vi "挥发酚通讯.vi"() -> ()   [LabVIEW 2022 SP3, in "挥发酚.lvlib"]
uses:
  <vilib>/Utility/config.llb/Write Key (String).vi
  <vilib>/Plasmionique/MB Master/MB_Master/MB_Master.lvclass
  <vilib>/Utility/config.llb/NI_LVConfig.lvlib
  <vilib>/Plasmionique/MB Master/MB Master.lvlib
  <userlib>/_OpenG.lib/variantconfig/variantconfig.llb/openg_variant_configuration_file.lvlib
  <vilib>/ptbypt/NI_PtbyPt.lvlib
panel:
  out "状态告警区":T1 {"工作状态" items=["空闲"=0, "水样测试"=1, "标样核查"=2, "零点核查"=3, "跨度核查"=4, "空白测试"=5, "平行样测试"=6, "加标回收"=7, "空白校准"=8, "标样校准"=9, "标定"=19, "初始化（清洗）"=10, "标样1测量"=28, "标样2测量"=29, "故障"=30, "异常处理"=31, "初始装液"=32, "其他"=33]; "告警代码" items=["无告警", "缺试剂告警", "缺水样告警", "缺蒸馏水告警", "缺标液告警", "仪表漏液告警", "标定异常告警", "超量程告警", "加热异常", "低试剂预警", "超上限告警", "超下限告警", "仪表内部其他异常", "滴定异常告警", "电极异常告警", "量程切换告警", "参数设置告警", "PH电极电位异常", "电导率电极异常", "浊度光度异常", "溶解氧电极异常", "溶解氧光强异常", "温度异常告警", "PH异常告警", "溶解氧异常告警", "电导率异常告警", "浊度异常告警", "叶绿素异常告警", "藻密度异常告警", "蓝绿藻异常告警", "ORP异常告警", "氨氮异常告警", "清洁刷异常告警", "SD卡异常告警", "蓝牙异常告警", "Wifi异常告警", "流程异常告警"]; "故障代码" items=["无故障", "电机故障", "温度故障", "通讯故障", "滴定故障"]}
  out "控制命令 2":u16[](array[numeric]) format="%xH"
  out "测量数据区":T2 {"单位" items=["ug/L", "mg/L", "ppm", "mg/m3", "cm", "ppb", "ug/m3", "%", "nmol/mol", "umol/mol", "MPN/L", "MPN/100ml", "ng/m3", "NTU", "无量纲", "ms/cm", "us/cm", "℃", "mV", "万个/L"]}
  out "状态告警区":u16[](array[numeric])
  out "测量数据区":u16[](array[numeric])
  out "序列号":string
  out "status":bool
  out "关键参数区":T3
  in  "读关键参数区":bool
  in  "读状态告警区":bool
  in  "读测量数据区":bool
  in  "站号":u16(ring) items=["CODMn"=21, "氨氮"=3, "挥发酚"=1]
  in  "停止":bool
  in  "启动":bool
  in  "控制命令":u16(ring) items=["启动测量"=1, "标样核查"=2, "零点核查"=3, "跨度核查"=4, "空白测试"=5, "平行样测试"=6, "加标回收"=7, "空白校准"=8, "标样校准"=9, "初始化（清洗）"=10, "停止测试"=11, "仪器重启"=12, "校时"=13, "模式设置"=14, "测量间隔设置"=15]
  in  "控制命令参数":u16[](array[numeric]) format="%04xH"
  in  "VISA Resource":refnum<visa-resource-name>
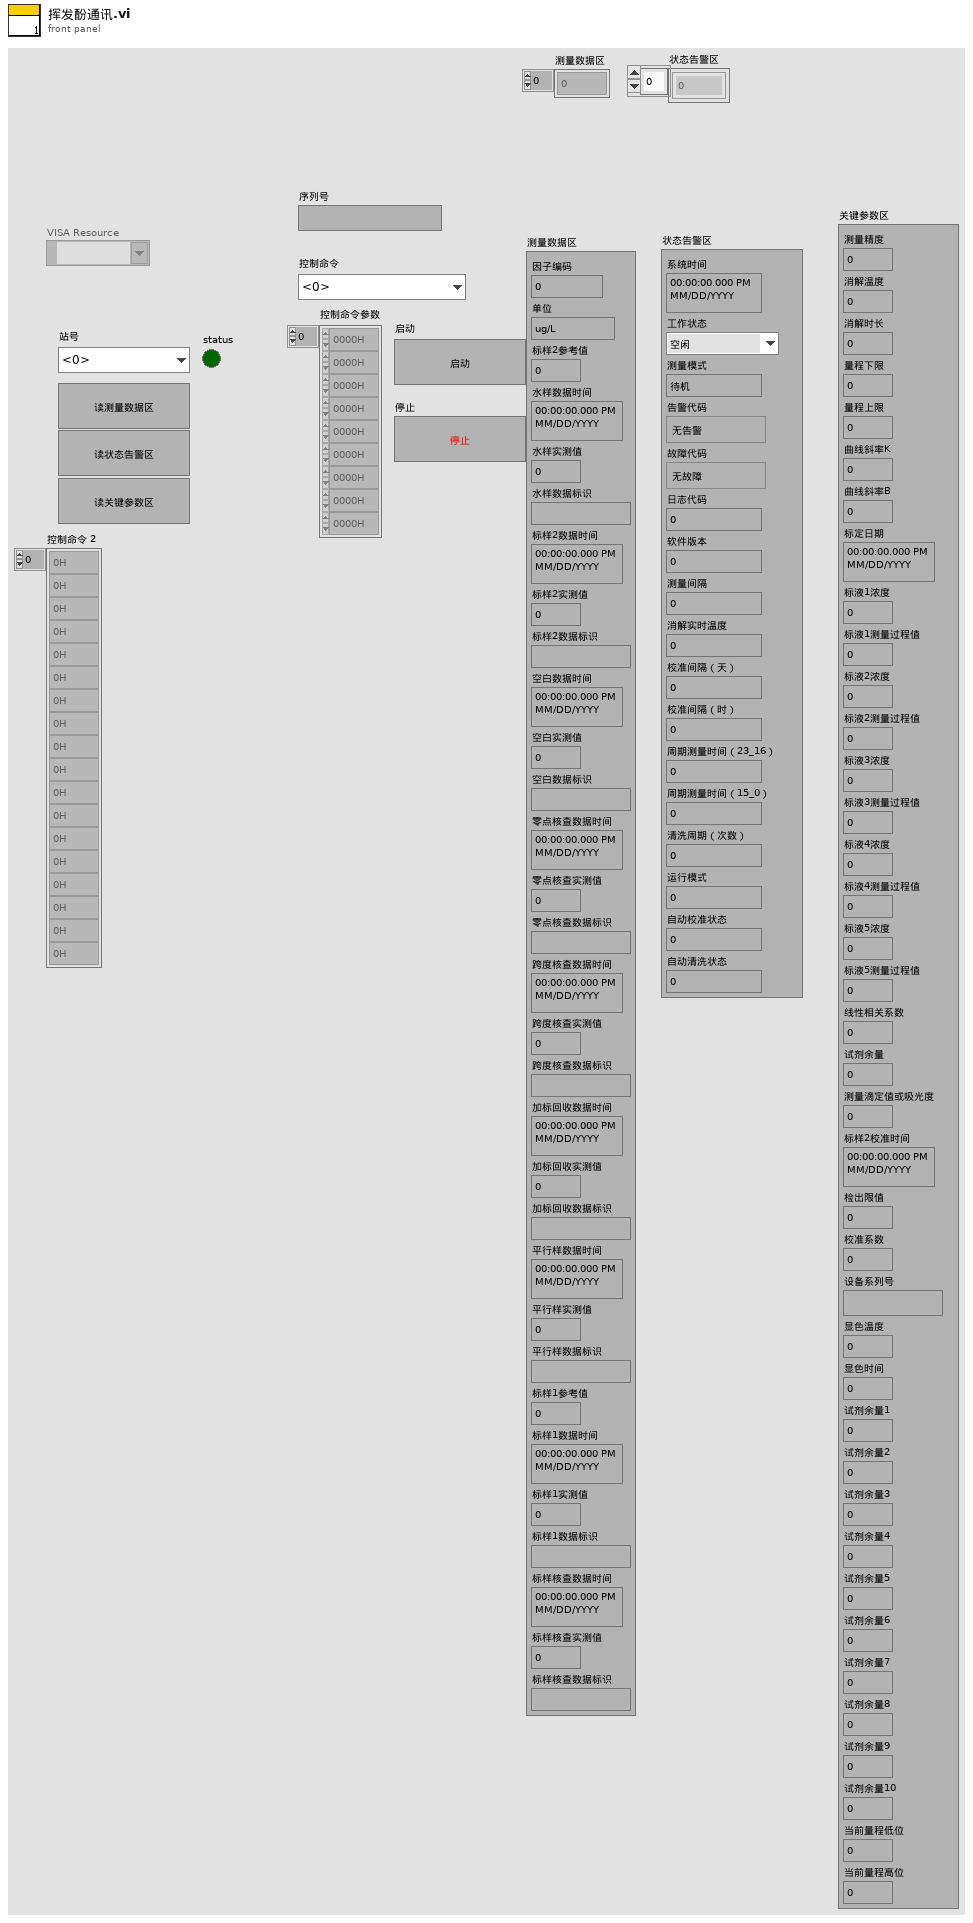
[diagram p1: front panel]
types:
  T1 = cluster{"系统时间":timestamp, "工作状态":u16, "测量模式":enum16{"待机", "连续模式", "周期模式", "定点模式", "受控模式", "手动模式"}, "告警代码":u16, "故障代码":u16, "日志代码":u16, "软件版本":u16, "测量间隔":u16, "消解实时温度":dbl, "校准间隔（天）":u16, "校准间隔（时）":u16, "周期测量时间（23_16）":u16, "周期测量时间（15_0）":u16, "清洗周期（次数）":u16, "运行模式":u16, "自动校准状态":u16, "自动清洗状态":u16}
  T2 = cluster{"因子编码":u32, "单位":u16, "标样2参考值":sgl, "水样数据时间":timestamp, "水样实测值":sgl, "水样数据标识":string, "标样2数据时间":timestamp, "标样2实测值":sgl, "标样2数据标识":string, "空白数据时间":timestamp, "空白实测值":sgl, "空白数据标识":string, "零点核查数据时间":timestamp, "零点核查实测值":sgl, "零点核查数据标识":string, "跨度核查数据时间":timestamp, "跨度核查实测值":sgl, "跨度核查数据标识":string, "加标回收数据时间":timestamp, "加标回收实测值":sgl, "加标回收数据标识":string, "平行样数据时间":timestamp, "平行样实测值":sgl, "平行样数据标识":string, "标样1参考值":sgl, "标样1数据时间":timestamp, "标样1实测值":sgl, "标样1数据标识":string, "标样核查数据时间":timestamp, "标样核查实测值":sgl, "标样核查数据标识":string}
  T3 = cluster{"测量精度":u16, "消解温度":u16, "消解时长":u16, "量程下限":sgl, "量程上限":sgl, "曲线斜率K":sgl, "曲线斜率B":sgl, "标定日期":timestamp, "标液1浓度":sgl, "标液1测量过程值":sgl, "标液2浓度":sgl, "标液2测量过程值":sgl, "标液3浓度":sgl, "标液3测量过程值":sgl, "标液4浓度":sgl, "标液4测量过程值":sgl, "标液5浓度":sgl, "标液5测量过程值":sgl, "线性相关系数":sgl, "试剂余量":u32, "测量滴定值或吸光度":sgl, "标样2校准时间":timestamp, "检出限值":sgl, "校准系数":sgl, "设备系列号":string, "显色温度":u16, "显色时间":u16, "试剂余量1":u16, "试剂余量2":u16, "试剂余量3":u16, "试剂余量4":u16, "试剂余量5":u16, "试剂余量6":u16, "试剂余量7":u16, "试剂余量8":u16, "试剂余量9":u16, "试剂余量10":u16, "当前量程低位":sgl, "当前量程高位":sgl}
  T4 = cluster{"测量模式":enum16{"水样测量", "标样核查", "零点核查", "跨度核查", "空白测试", "加标回收", "平行样", "校零", "校标"}}
  T5 = typedef "NI_LVConfig.lvlib/Config Data RefNum.ctl" = refnum<k1>
  T6 = cluster{"站号":u16, "量程切换":enum32{"H", "L", "AUTO"}, "控制命令":u16, "模式设置":enum16{"待机", "连续模式", "周期模式", "定点模式", "受控模式", "手动模式"}, "测量间隔":u16}
  T7 = enum16{"水样测量", "标样核查", "零点核查", "跨度核查", "空白测试", "加标回收", "平行样", "校零", "校标"}
  T8 = enum8{"Enabled", "Disabled", "Disabled and Grayed Out"}
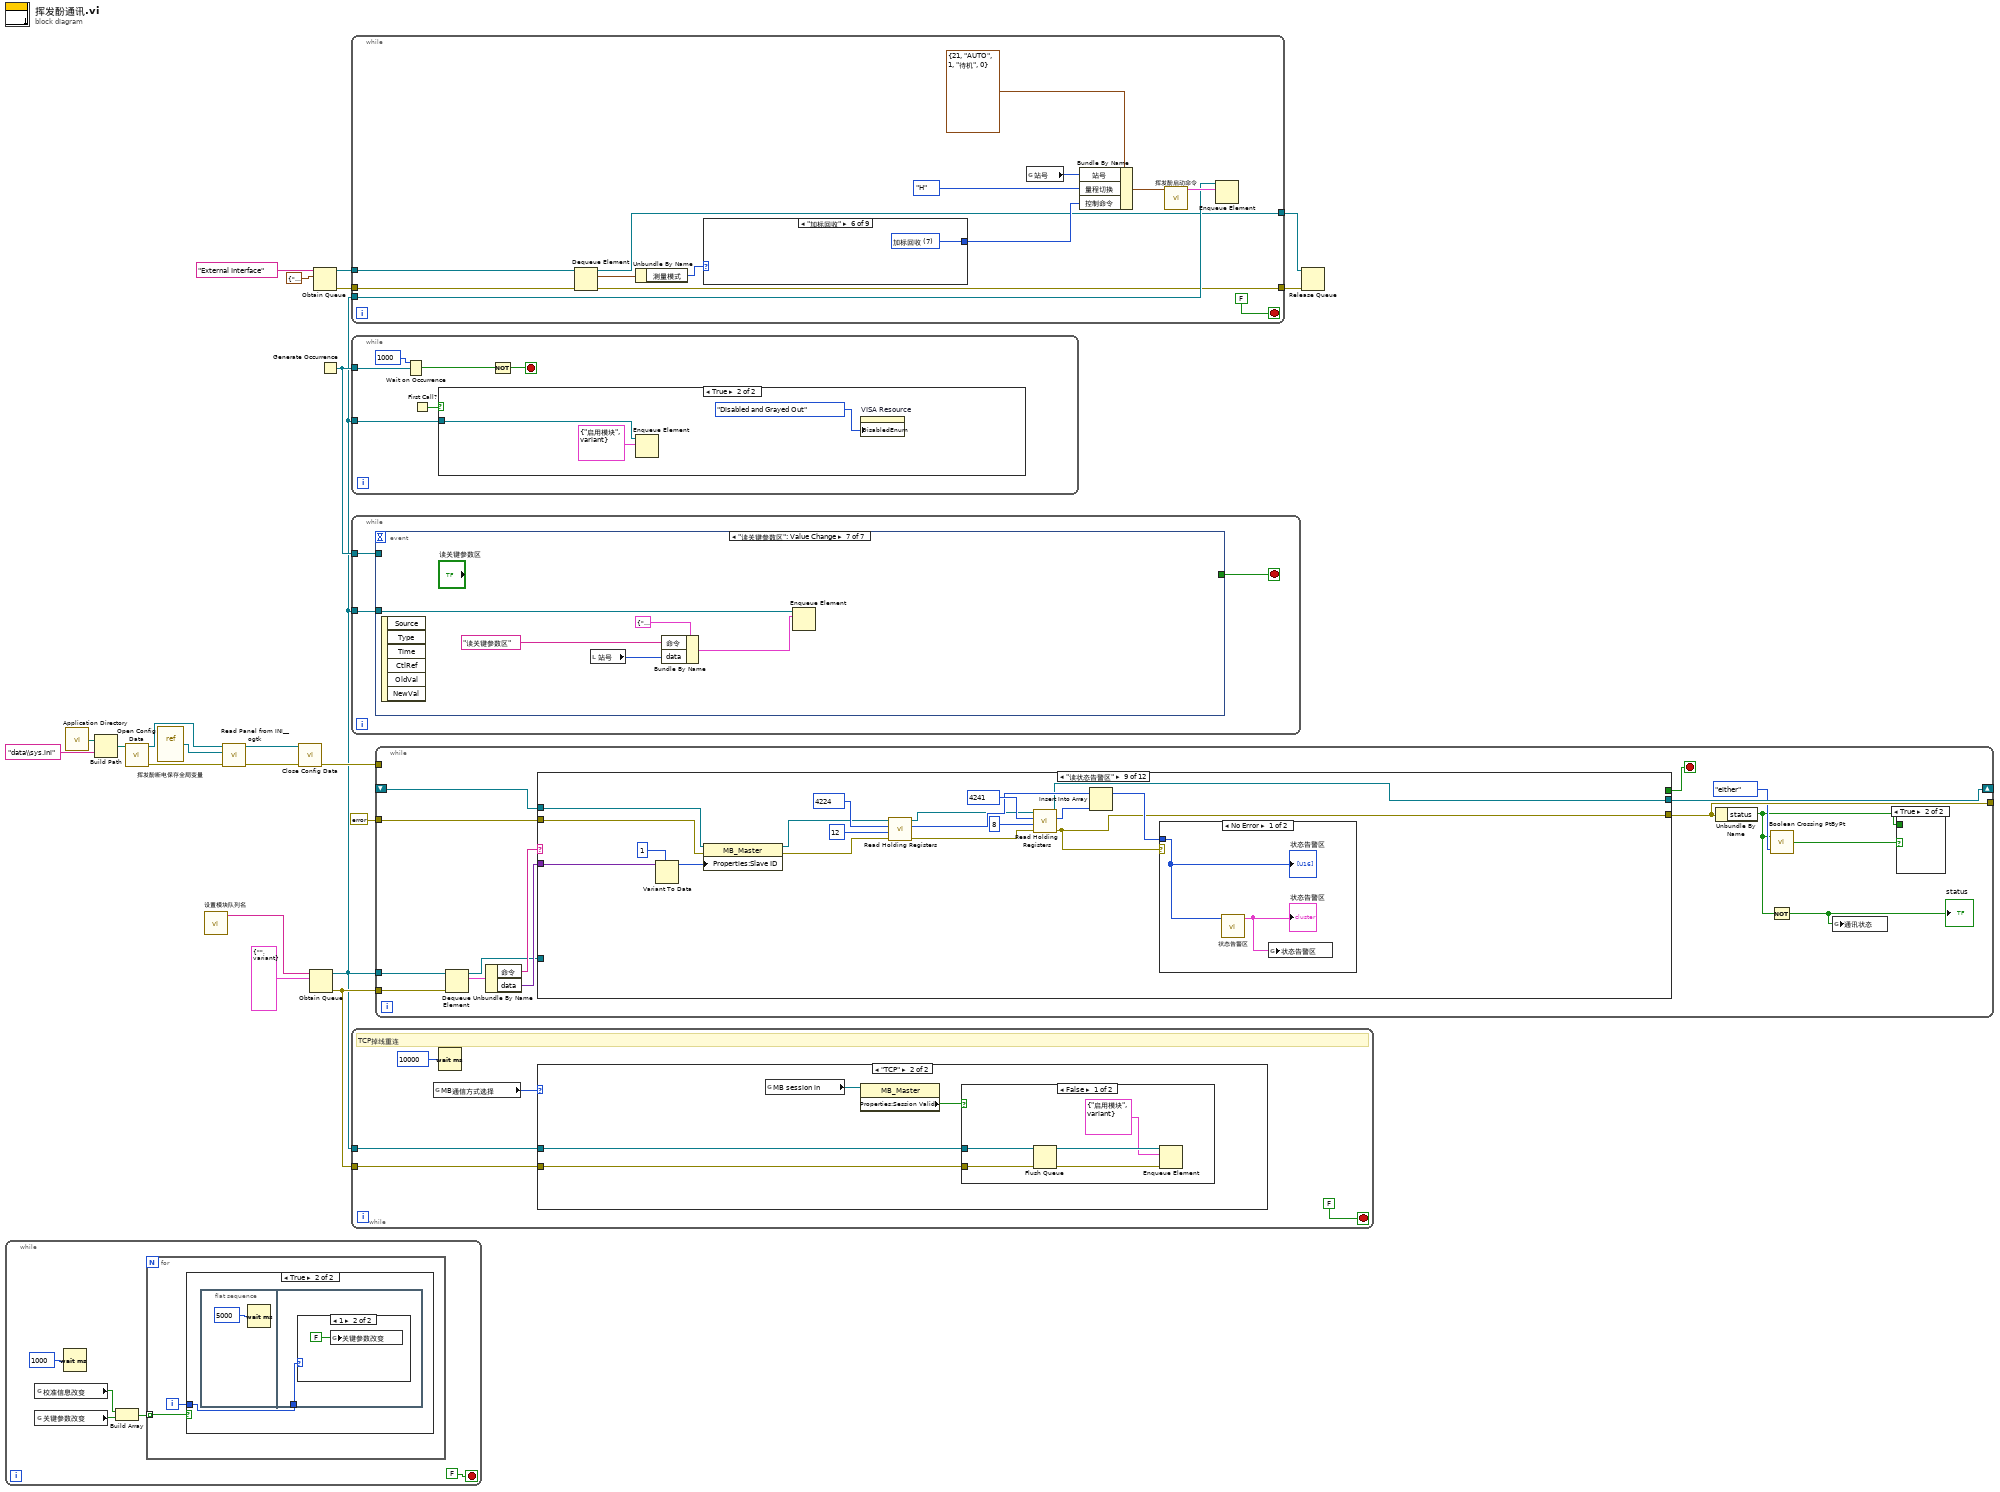
[diagram p0: block diagram]
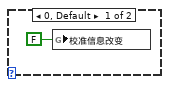
[diagram p3: hidden frame]
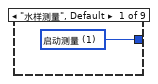
[diagram p4: hidden frame]
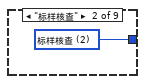
[diagram p5: hidden frame]
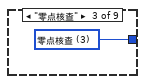
[diagram p6: hidden frame]
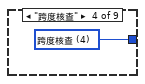
[diagram p7: hidden frame]
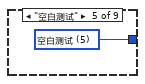
[diagram p8: hidden frame]
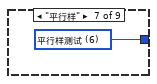
[diagram p9: hidden frame]
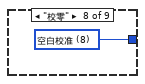
[diagram p10: hidden frame]
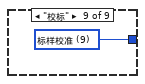
[diagram p11: hidden frame]
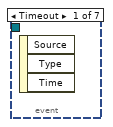
[diagram p15: hidden frame]
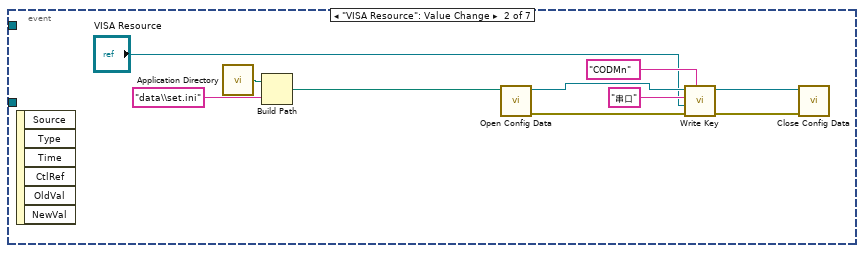
[diagram p16: hidden frame]
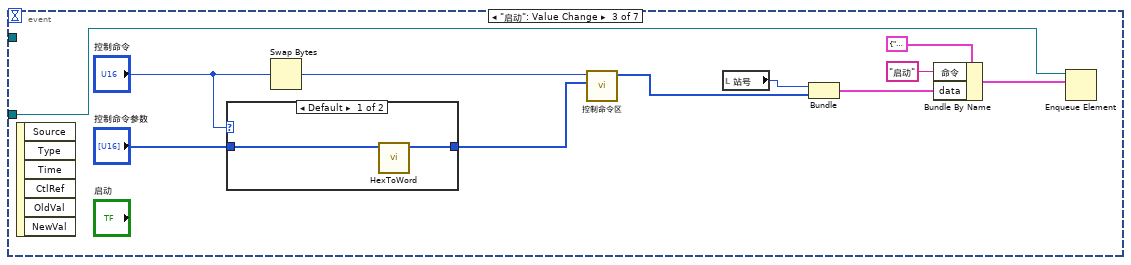
[diagram p17: hidden frame]
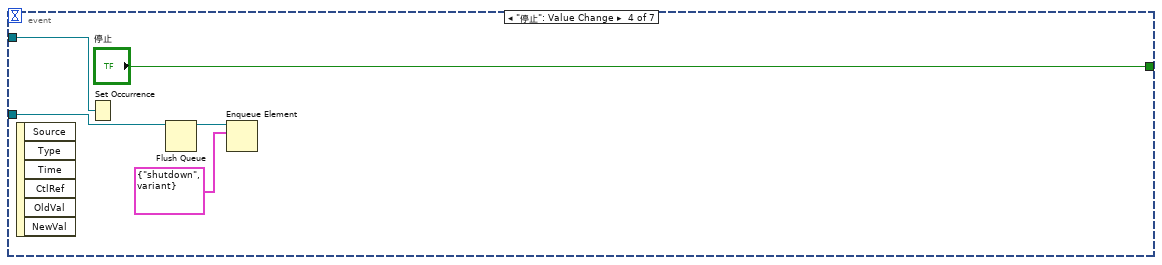
[diagram p19: hidden frame]
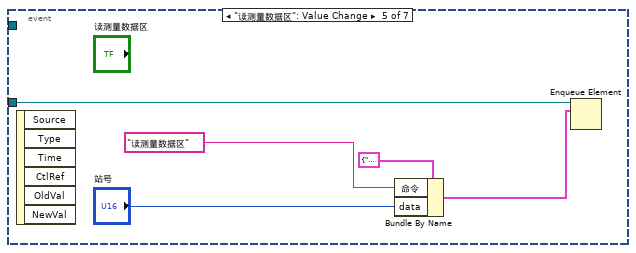
[diagram p20: hidden frame]
diagram:
  n1 = while {
    stop <- FALSE stop-if-true
    n2 = global read "挥发酚断电保存全局变量.vi" "校准信息改变"() -> (w24:bool)
    n3 = global read "挥发酚断电保存全局变量.vi" "关键参数改变"() -> (w23:bool)
    n4 = Wait (ms)(milliseconds to wait=u32 1000 ("等待时间（毫秒）")) -> ()  [unwired: 1 out]
    n5 = Build Array(w24, w23) -> (w22:bool[])
    n6 = for {
      tunnel: w22 -> [w28] mode=indexing
      i -> [w27]
      n7 = case shown="True" w28 {
        tunnel: w27 -> [_ w29]
        frame False {
        }
        frame True {
          n8 = flat-sequence {
            tunnel: w29 -> [w31]
            frame #0 {
              n9 = Wait (ms)(milliseconds to wait=u32 5000 ("等待时间（毫秒）")) -> ()  [unwired: 1 out]
            }
            frame #1 {
              n10 = case shown="1" w31 {
                frame 0, Default {
                  n11 = global write "挥发酚断电保存全局变量.vi" "校准信息改变"(FALSE ("关键参数改变")) -> ()
                }
                frame 1 {
                  n12 = global write "挥发酚断电保存全局变量.vi" "关键参数改变"(FALSE ("关键参数改变")) -> ()
                }
              }
            }
          }
        }
      }
    }
  }
  n13 = call <vilib>:"Application Directory.vi"() -> ("Application Directory"=w2:path)
  n14 = Build Path(base path=w2, name or relative path="data\\sys.ini" ("名称或相对路径")) -> (appended path=w11:path)
  n15 = call <vilib>:"Open Config Data.vi"("configuration file path"=w11) -> ("error out"=w17:errorcluster, "refnum"=w14:T5)  [unwired: 8 in, 1 out]
  n16 = vi-ref "挥发酚断电保存全局变量.vi"() -> (w15:refnum<vi>)
  n17 = call "设置模块队列名.vi"() -> ("Msg"=w3:string)  [unwired: 11 in]
  n18 = call <userlib>:"Read Panel from INI__ogtk.vi"("error in (no error)"=w17, "VI ref"=w15, "refnum"=w14) -> ("error out"=w18:errorcluster, "refnum out"=w16:T5)  [unwired: 7 in]
  n19 = call <vilib>:"Close Config Data.vi"("error in (no error)"=w18, "refnum"=w16) -> ("error out"=w13:errorcluster)  [unwired: 8 in, 1 out]
  n20 = Obtain Queue(name (unnamed)=w3, element data type=cluster{"命令":string, "data":variant} {"命令"="", "data"=variant}) -> (queue out=w7:refnum<queue>, error out=w12:errorcluster)  [unwired: 3 in, 1 out]
  n21 = Obtain Queue(name (unnamed)="External Interface" ("名称（未命名）"), element data type=T4 {"测量模式"=enum."水样测量"} ("元素")) -> (queue out=w9:refnum<queue>, error out=w8:errorcluster)  [unwired: 3 in, 1 out]
  n22 = Generate Occurrence() -> (w19:refnum<k4>)
  n23 = while {
    tunnel: w9 -> [w47]
    tunnel: w8 -> [w46]
    tunnel: w7 -> [w38]
    tunnel: [w37] -> w6
    tunnel: [w36] -> w5
    stop <- FALSE stop-if-true
    n24 = Dequeue Element(queue=w47, error in (no error)=w46) -> (queue out=w37:refnum<queue>, element=w41:T4, error out=w36:errorcluster)  [unwired: 1 in, 1 out]
    n25 = Unbundle By Name(w41) -> ("测量模式"=w40:T7)
    n26 = case shown="\"加标回收\"" w40 {
      tunnel: [w48 w49 w50 w51 w52 w53 w54 w55 w56] -> w39
      frame "水样测量", Default {
        w48 = u16 1 items=["启动测量"=1, "标样核查"=2, "零点核查"=3, "跨度核查"=4, "空白测试"=5, "平行样测试"=6, "加标回收"=7, "空白校准"=8, "标样校准"=9, "初始化（清洗）"=10, "停止测试"=11, "仪器重启"=12, "校时"=13, "模式设置"=14, "测量间隔设置"=15, "调试"=22, "填充管路"=30, "清洗管路"=31, "清洗反应杯"=32] ("控制命令")
      }
      frame "标样核查" {
        w49 = u16 2 items=["启动测量"=1, "标样核查"=2, "零点核查"=3, "跨度核查"=4, "空白测试"=5, "平行样测试"=6, "加标回收"=7, "空白校准"=8, "标样校准"=9, "初始化（清洗）"=10, "停止测试"=11, "仪器重启"=12, "校时"=13, "模式设置"=14, "测量间隔设置"=15, "调试"=22, "填充管路"=30, "清洗管路"=31, "清洗反应杯"=32] ("控制命令")
      }
      frame "零点核查" {
        w50 = u16 3 items=["启动测量"=1, "标样核查"=2, "零点核查"=3, "跨度核查"=4, "空白测试"=5, "平行样测试"=6, "加标回收"=7, "空白校准"=8, "标样校准"=9, "初始化（清洗）"=10, "停止测试"=11, "仪器重启"=12, "校时"=13, "模式设置"=14, "测量间隔设置"=15, "调试"=22, "填充管路"=30, "清洗管路"=31, "清洗反应杯"=32] ("控制命令")
      }
      frame "跨度核查" {
        w51 = u16 4 items=["启动测量"=1, "标样核查"=2, "零点核查"=3, "跨度核查"=4, "空白测试"=5, "平行样测试"=6, "加标回收"=7, "空白校准"=8, "标样校准"=9, "初始化（清洗）"=10, "停止测试"=11, "仪器重启"=12, "校时"=13, "模式设置"=14, "测量间隔设置"=15, "调试"=22, "填充管路"=30, "清洗管路"=31, "清洗反应杯"=32] ("控制命令")
      }
      frame "空白测试" {
        w52 = u16 5 items=["启动测量"=1, "标样核查"=2, "零点核查"=3, "跨度核查"=4, "空白测试"=5, "平行样测试"=6, "加标回收"=7, "空白校准"=8, "标样校准"=9, "初始化（清洗）"=10, "停止测试"=11, "仪器重启"=12, "校时"=13, "模式设置"=14, "测量间隔设置"=15, "调试"=22, "填充管路"=30, "清洗管路"=31, "清洗反应杯"=32] ("控制命令")
      }
      frame "加标回收" {
        w53 = u16 7 items=["启动测量"=1, "标样核查"=2, "零点核查"=3, "跨度核查"=4, "空白测试"=5, "平行样测试"=6, "加标回收"=7, "空白校准"=8, "标样校准"=9, "初始化（清洗）"=10, "停止测试"=11, "仪器重启"=12, "校时"=13, "模式设置"=14, "测量间隔设置"=15, "调试"=22, "填充管路"=30, "清洗管路"=31, "清洗反应杯"=32] ("控制命令")
      }
      frame "平行样" {
        w54 = u16 6 items=["启动测量"=1, "标样核查"=2, "零点核查"=3, "跨度核查"=4, "空白测试"=5, "平行样测试"=6, "加标回收"=7, "空白校准"=8, "标样校准"=9, "初始化（清洗）"=10, "停止测试"=11, "仪器重启"=12, "校时"=13, "模式设置"=14, "测量间隔设置"=15, "调试"=22, "填充管路"=30, "清洗管路"=31, "清洗反应杯"=32] ("控制命令")
      }
      frame "校零" {
        w55 = u16 8 items=["启动测量"=1, "标样核查"=2, "零点核查"=3, "跨度核查"=4, "空白测试"=5, "平行样测试"=6, "加标回收"=7, "空白校准"=8, "标样校准"=9, "初始化（清洗）"=10, "停止测试"=11, "仪器重启"=12, "校时"=13, "模式设置"=14, "测量间隔设置"=15, "调试"=22, "填充管路"=30, "清洗管路"=31, "清洗反应杯"=32] ("控制命令")
      }
      frame "校标" {
        w56 = u16 9 items=["启动测量"=1, "标样核查"=2, "零点核查"=3, "跨度核查"=4, "空白测试"=5, "平行样测试"=6, "加标回收"=7, "空白校准"=8, "标样校准"=9, "初始化（清洗）"=10, "停止测试"=11, "仪器重启"=12, "校时"=13, "模式设置"=14, "测量间隔设置"=15, "调试"=22, "填充管路"=30, "清洗管路"=31, "清洗反应杯"=32] ("控制命令")
      }
    }
    n27 = global read "挥发酚断电保存全局变量.vi" "站号"() -> (w42:u16)
    n28 = Bundle By Name(cluster=T6 {"站号"=21, "量程切换"=enum."AUTO", "控制命令"=1, "模式设置"=enum."待机", "测量间隔"=0} ("参数"), "站号"=w42, "量程切换"=enum32{"H", "L", "AUTO"}."H", "控制命令"=w39) -> (w43:T6)
    n29 = call "挥发酚启动命令.vi"("参数"=w43) -> ("启动命令"=w45:cluster{"命令":string, "data":variant})  [unwired: 10 in]
    n30 = Enqueue Element(queue=w38, element=w45) -> ()  [unwired: 2 in, 3 out]
  }
  n31 = while {
    tunnel: w19 -> [w62]
    tunnel: w7 -> [w58]
    stop <- w59 stop-if-true
    n32 = Wait on Occurrence(2:w62, 3:1000 ("毫秒超时(-1)")) -> (0:w60:bool)  [unwired: 1 in]
    n33 = First Call?() -> (First Call?: T/F=w57:bool)
    n34 = case shown="True" w57 {
      tunnel: w58 -> [_ w64]
      frame False {
      }
      frame True {
        n35 = Enqueue Element(queue=w64, element=cluster{"命令":string, "data":variant} {"命令"="启用模块", "data"=variant} ("元素")) -> ()  [unwired: 2 in, 3 out]
        n36 = property on="VISA Resource" class="VISAName"("DisabledEnum"=T8."Disabled and Grayed Out" ("禁用")) -> ()  [unwired: 2 in, 2 out]
      }
    }
    n37 = Not(x=w60) -> (.not. x?=w59:bool)
  }
  n38 = while {
    tunnel: w7 -> [w68]
    tunnel: w19 -> [w66]
    stop <- w67 stop-if-true
    n39 = event shown="[6] \"读关键参数区\": Value Change" {
      selector: _ -> [_ _ _ _ _ _ _]
      dyn-events: _ -> [_ _ _ _ _ _ _]
      timeout: _ -> [_ _ _ _ _ _ _]
      tunnel: w68 -> [_ _ w89 w96 w102 w107 w112]
      tunnel: [_ _ _ "停止" _ _ _] -> w67
      tunnel: w66 -> [_ _ _ w93 _ _ _]
      event Timeout {
        n40 = event-data() -> ()  [unwired: 1 in, 3 out]
      }
      event "VISA Resource": Value Change {
        n41 = event-data() -> ()  [unwired: 1 in, 6 out]
        n42 = call <vilib>:"Application Directory.vi"() -> ("Application Directory"=w71:path)
        n43 = Build Path(base path=w71, name or relative path="data\\set.ini" ("名称或相对路径")) -> (appended path=w72:path)
        n44 = call <vilib>:"Open Config Data.vi"("configuration file path"=w72) -> ("error out"=w78:errorcluster, "refnum"=w77:T5)  [unwired: 8 in, 1 out]
        n45 = call-poly <vilib>:"Write Key.vi"("section"="CODMn", "error in (no error)"=w78, "value"="VISA Resource", "key"="串口", "refnum"=w77) -> ("error out"=w74:errorcluster, "refnum out"=w70:T5)  [unwired: 4 in, 1 out]
        n46 = call <vilib>:"Close Config Data.vi"("error in (no error)"=w74, "refnum"=w70) -> ()  [unwired: 8 in, 2 out]
      }
      event "启动": Value Change {
        n47 = event-data() -> ()  [unwired: 1 in, 6 out]
        n48 = case shown="Default" "控制命令" {
          tunnel: "控制命令参数" -> [w91 w92]
          tunnel: [w90 w92] -> w79
          frame Default {
            n49 = call "HexToWord.vi"("数组"=w91) -> ("WORD"=w90:u16[])  [unwired: 10 in]
          }
          frame 13 {
          }
        }
        n50 = Swap Bytes(anything="控制命令") -> (byte swapped=w82:u16)
        n51 = call "控制命令区.vi"("控制命令参数"=w79, "控制命令"=w82) -> ("控制命令"=w85:u16[])  [unwired: 9 in]
        n52 = local read "站号"() -> (w84:u16)
        n53 = Bundle("站号"=w84, "控制命令"=w85) -> (w83:cluster{"站号":u16, "控制命令":u16[]})  [unwired: 1 in]
        n54 = Bundle By Name(cluster=cluster{"命令":string, "data":variant} {"命令"="", "data"=variant} ("元素"), "命令"="启动", "data"=w83) -> (w87:cluster{"命令":string, "data":variant})
        n55 = Enqueue Element(queue=w89, element=w87) -> ()  [unwired: 2 in, 3 out]
      }
      event "停止": Value Change {
        n56 = event-data() -> ()  [unwired: 1 in, 6 out]
        n57 = Set Occurrence(w93) -> ()
        n58 = Flush Queue(queue=w96) -> (queue out=w95:refnum<queue>)  [unwired: 1 in, 2 out]
        n59 = Enqueue Element(queue=w95, element=cluster{"命令":string, "data":variant} {"命令"="shutdown", "data"=variant} ("元素")) -> ()  [unwired: 2 in, 3 out]
      }
      event "读测量数据区": Value Change {
        n60 = event-data() -> ()  [unwired: 1 in, 6 out]
        n61 = Bundle By Name(cluster=cluster{"命令":string, "data":variant} {"命令"="", "data"=variant} ("元素"), "命令"="读测量数据区", "data"="站号") -> (w100:cluster{"命令":string, "data":variant})
        n62 = Enqueue Element(queue=w102, element=w100) -> ()  [unwired: 2 in, 3 out]
      }
      event "读状态告警区": Value Change {
        n63 = event-data() -> ()  [unwired: 1 in, 6 out]
        n64 = local read "站号"() -> (w103:u16)
        n65 = Bundle By Name(cluster=cluster{"命令":string, "data":variant} {"命令"="", "data"=variant} ("元素"), "命令"="读状态告警区", "data"=w103) -> (w105:cluster{"命令":string, "data":variant})
        n66 = Enqueue Element(queue=w107, element=w105) -> ()  [unwired: 2 in, 3 out]
      }
      event "读关键参数区": Value Change {
        n67 = event-data() -> ()  [unwired: 1 in, 6 out]
        n68 = local read "站号"() -> (w108:u16)
        n69 = Bundle By Name(cluster=cluster{"命令":string, "data":variant} {"命令"="", "data"=variant} ("元素"), "命令"="读关键参数区", "data"=w108) -> (w110:cluster{"命令":string, "data":variant})
        n70 = Enqueue Element(queue=w112, element=w110) -> ()  [unwired: 2 in, 3 out]
      }
    }
  }
  n71 = while "While循环" {
    tunnel: w7 -> [w115]
    tunnel: w12 -> [w114]
    stop <- FALSE stop-if-true
    # "TCP掉线重连"
    n72 = global read "挥发酚断电保存全局变量.vi" "MB通信方式选择"() -> (w113:enum16{"串口", "TCP"})
    n73 = Wait (ms)(milliseconds to wait=u32 10000 ("等待时间（毫秒）")) -> ()  [unwired: 1 out]
    n74 = case shown="\"TCP\"" w113 {
      tunnel: w115 -> [_ w120]
      tunnel: w114 -> [_ w119]
      frame "串口", Default {
      }
      frame "TCP" {
        n75 = global read "VAR挥发酚全局变量.vi" "MB session in"() -> (w118:refnum<class "MB_Master.lvclass">)
        n76 = property class="MB_Master"(reference=w118) -> ("Properties:Session Valid"=w121:bool)  [unwired: 1 in, 2 out]
        n77 = case shown="False" w121 {
          tunnel: w120 -> [w124 _]
          tunnel: w119 -> [w123 _]
          frame False {
            n78 = Flush Queue(queue=w124, error in (no error)=w123) -> (queue out=w126:refnum<queue>, error out=w125:errorcluster)  [unwired: 1 out]
            n79 = Enqueue Element(queue=w126, element=cluster{"命令":string, "data":variant} {"命令"="启用模块", "data"=variant} ("元素"), error in (no error)=w125) -> ()  [unwired: 1 in, 3 out]
          }
          frame True {
          }
        }
      }
    }
  }
  n80 = while {
    tunnel: w7 -> [w141]
    tunnel: w12 -> [w140]
    shift-right: [w138] -> _
    shift-left: _ -> [w137]
    tunnel: errorcluster {"status"=FALSE, "code"=0, "source"=""} ("error out") -> [w136]
    tunnel: [w131] -> _
    tunnel: w13 -> [_]
    stop <- w139 stop-if-true
    n81 = Dequeue Element(queue=w141, error in (no error)=w140) -> (queue out=w132:refnum<queue>, element=w134:cluster{"命令":string, "data":variant})  [unwired: 1 in, 2 out]
    n82 = Unbundle By Name(w134) -> ("命令"=w135:string, "data"=w133:variant)
    n83 = case shown="\"读状态告警区\"" w135 {
      tunnel: w133 -> [_ _ _ w160 w171 w188 w200 w209 w227 w266 w280 _]
      tunnel: w132 -> [_ _ _ _ _ _ _ _ _ _ _ w293]
      tunnel: [_ _ _ _ _ _ _ _ _ _ _ TRUE] -> w139
      tunnel: [w142 w145 w147 w163 w174 w190 w202 w214 w221 w239 w287 w289] -> w138
      tunnel: [w143 w144 w148 w162 w173 w189 w201 w203 w217 w237 w288 w290] -> w131
      tunnel: w137 -> [w142 _ w147 w159 w170 w187 w199 w208 w230 w269 w283 w289]
      tunnel: w136 -> [w143 _ w150 w156 w167 w184 w196 w206 w231 w270 w284 w291]
      frame Default {
      }
      frame "启用模块" {
        n84 = call "MB_api.vi"("STEP"=enum16{"open", "read", "write", "close"}."open") -> ("error out"=w144:errorcluster, "MB session out"=w145:refnum<class "MB_Master.lvclass">)  [unwired: 8 in, 1 out]
        n85 = global write "VAR挥发酚全局变量.vi" "MB session in"(w145) -> ()
      }
      frame "停用模块" {
        n86 = call-dynamic "Close Session.vi"("error in (no error)"=w150, "MB session in"=w147) -> ("error out"=w149:errorcluster)  [unwired: 9 in]
        n87 = call <vilib>:"Clear Errors.vi"("error in (no error)"=w149) -> ("error out"=w148:errorcluster)  [unwired: 5 in, 1 out]
      }
      frame "启动" {
        n88 = Variant To Data(type=cluster{"站号":u16, "控制命令":u16[]} {"站号"=0, "控制命令"=[]} ("输出簇"), Variant=w160) -> (data=w154:cluster{"站号":u16, "控制命令":u16[]})  [unwired: 1 in, 1 out]
        n89 = Unbundle By Name(w154) -> ("站号"=w153:u16, "控制命令"=w151:u16[])
        n90 = property class="MB_Master"(reference=w159, error in=w156, "Properties:Slave ID"=w153) -> (reference out=w158:refnum<class "MB_Master.lvclass">, error out=w157:errorcluster)
        n91 = Index Array(array=w151) -> (element=w152:u16)  [unwired: 1 in]
        n92 = global write "VAR挥发酚全局变量.vi" "控制命令"(w152) -> ()
        n93 = call <vilib>:"Write Multiple Registers.vi"("error in (no error)"=w157, "values"=w151, "starting address"=u16 4608, "MB session in"=w158) -> ("error out"=w162:errorcluster, "MB session out"=w163:refnum<class "MB_Master.lvclass">)  [unwired: 6 in]
      }
      frame "盲样测试" {
        n94 = Variant To Data(type=0, Variant=w171) -> (data=w164:i32)  [unwired: 1 in, 1 out]
        n95 = property class="MB_Master"(reference=w170, error in=w167, "Properties:Slave ID"=w164) -> (reference out=w169:refnum<class "MB_Master.lvclass">, error out=w168:errorcluster)
        n96 = case shown="Default" w164 {
          tunnel: [u16[] [] ("values") u16[] [33539, 0] ("values") u16[] [23555, 0] ("values")] -> w166
          frame Default {
          }
          frame 1 {
            # "总磷盲样测试命令"
          }
          frame 3 {
            # "氨氮盲样测试"
          }
        }
        n97 = call <vilib>:"Write Multiple Registers.vi"("error in (no error)"=w168, "values"=w166, "starting address"=u16 24592, "MB session in"=w169) -> ("error out"=w173:errorcluster, "MB session out"=w174:refnum<class "MB_Master.lvclass">)  [unwired: 6 in]
      }
      frame "debug" {
        n98 = Variant To Data(type=cluster{"站号":u16, "控制命令":u16[]} {"站号"=0, "控制命令"=[]} ("输出簇"), Variant=w188) -> (data=w182:cluster{"站号":u16, "控制命令":u16[]})  [unwired: 1 in, 1 out]
        n99 = Unbundle By Name(w182) -> ("站号"=w181:u16, "控制命令"=w179:u16[])
        "控制命令 2" <- w179
        n100 = property class="MB_Master"(reference=w187, error in=w184, "Properties:Slave ID"=w181) -> (reference out=w186:refnum<class "MB_Master.lvclass">, error out=w185:errorcluster)
        n101 = Index Array(array=w179) -> (element=w180:u16)  [unwired: 1 in]
        n102 = global write "VAR挥发酚全局变量.vi" "控制命令"(w180) -> ()
        n103 = call <vilib>:"Write Multiple Registers.vi"("error in (no error)"=w185, "values"=w179, "starting address"=u16 24594, "MB session in"=w186) -> ("error out"=w189:errorcluster, "MB session out"=w190:refnum<class "MB_Master.lvclass">)  [unwired: 6 in]
      }
      frame "单步控制" {
        n104 = Variant To Data(type=cluster{"站号":u16, "控制命令":u16[]} {"站号"=0, "控制命令"=[]} ("输出簇"), Variant=w200) -> (data=w194:cluster{"站号":u16, "控制命令":u16[]})  [unwired: 1 in, 1 out]
        n105 = Unbundle By Name(w194) -> ("站号"=w193:u16, "控制命令"=w192:u16[])
        n106 = property class="MB_Master"(reference=w199, error in=w196, "Properties:Slave ID"=w193) -> (reference out=w198:refnum<class "MB_Master.lvclass">, error out=w197:errorcluster)
        n107 = call <vilib>:"Write Multiple Registers.vi"("error in (no error)"=w197, "values"=w192, "starting address"=u16 24610, "MB session in"=w198) -> ("error out"=w201:errorcluster, "MB session out"=w202:refnum<class "MB_Master.lvclass">)  [unwired: 6 in]
      }
      frame "读测量数据区" {
        n108 = Variant To Data(type=u8 1 ("Slave ID"), Variant=w209) -> (data=w210:u8)  [unwired: 1 in, 1 out]
        n109 = property class="MB_Master"(reference=w208, error in=w206, "Properties:Slave ID"=w210) -> (reference out=w207:refnum<class "MB_Master.lvclass">, error out=w205:errorcluster)
        n110 = call <vilib>:"Read Holding Registers.vi"("error in (no error)"=w205, "quantity"=u16 106, "starting address"=u16 4096, "MB session in"=w207) -> ("error out"=w203:errorcluster, "Registers"=w204:u16[], "MB session out"=w214:refnum<class "MB_Master.lvclass">)  [unwired: 5 in]
        n111 = case shown="No Error" w203 {
          tunnel: w204 -> [w216 _]
          frame No Error {
            n112 = call "测量数据区.vi"("数组"=w216) -> ("测量数据区"=w215:T2)  [unwired: 10 in]
            "测量数据区" <- w215
            n113 = global write "VAR挥发酚全局变量.vi" "测量数据区"(w215) -> ()
            "测量数据区" <- w216
          }
          frame Error {
          }
        }
      }
      frame "读状态告警区" {
        n114 = Variant To Data(type=u8 1 ("Slave ID"), Variant=w227) -> (data=w232:u8)  [unwired: 1 in, 1 out]
        n115 = property class="MB_Master"(reference=w230, error in=w231, "Properties:Slave ID"=w232) -> (reference out=w229:refnum<class "MB_Master.lvclass">, error out=w228:errorcluster)
        n116 = call <vilib>:"Read Holding Registers.vi"("error in (no error)"=w228, "quantity"=u16 12, "starting address"=u16 4224, "MB session in"=w229) -> ("error out"=w218:errorcluster, "Registers"=w223:u16[], "MB session out"=w222:refnum<class "MB_Master.lvclass">)  [unwired: 5 in]
        n117 = call <vilib>:"Read Holding Registers.vi"("error in (no error)"=w218, "quantity"=u16 8, "starting address"=u16 4241, "MB session in"=w222) -> ("error out"=w217:errorcluster, "Registers"=w220:u16[], "MB session out"=w221:refnum<class "MB_Master.lvclass">)  [unwired: 5 in]
        n118 = Insert Into Array(array=w223, new element=w220) -> (w219:u16[])  [unwired: 1 in]
        n119 = case shown="No Error" w217 {
          tunnel: w219 -> [w236 _]
          frame No Error {
            n120 = call "状态告警区.vi"("数组"=w236) -> ("状态告警区"=w235:T1)  [unwired: 10 in]
            "状态告警区" <- w235
            n121 = global write "VAR挥发酚全局变量.vi" "状态告警区"(w235) -> ()
            "状态告警区" <- w236
          }
          frame Error {
          }
        }
      }
      frame "读关键参数区" {
        n122 = Variant To Data(type=u8 1 ("Slave ID"), Variant=w266) -> (data=w264:u8)  [unwired: 1 in, 1 out]
        n123 = property class="MB_Master"(reference=w269, error in=w270, "Properties:Slave ID"=w264) -> (reference out=w268:refnum<class "MB_Master.lvclass">, error out=w267:errorcluster)
        n124 = call <vilib>:"Read Holding Registers.vi"("error in (no error)"=w267, "quantity"=u16 3, "starting address"=u16 4256, "MB session in"=w268) -> ("error out"=w262:errorcluster, "Registers"=w259:u16[], "MB session out"=w263:refnum<class "MB_Master.lvclass">)  [unwired: 5 in]
        n125 = call <vilib>:"Read Holding Registers.vi"("error in (no error)"=w262, "quantity"=u16 19, "starting address"=u16 4259, "MB session in"=w263) -> ("error out"=w249:errorcluster, "Registers"=w258:u16[], "MB session out"=w251:refnum<class "MB_Master.lvclass">)  [unwired: 5 in]
        n126 = call <vilib>:"Read Holding Registers.vi"("error in (no error)"=w249, "quantity"=u16 15, "starting address"=u16 4294, "MB session in"=w251) -> ("error out"=w244:errorcluster, "Registers"=w250:u16[], "MB session out"=w246:refnum<class "MB_Master.lvclass">)  [unwired: 5 in]
        n127 = call <vilib>:"Read Holding Registers.vi"("error in (no error)"=w244, "quantity"=u16 12, "starting address"=u16 4322, "MB session in"=w246) -> ("error out"=w238:errorcluster, "Registers"=w245:u16[], "MB session out"=w243:refnum<class "MB_Master.lvclass">)  [unwired: 5 in]
        n128 = Initialize Array(u16 0 ("quantity"), 16 ("维数大小")) -> (w254:u16[])
        n129 = call <vilib>:"Read Holding Registers.vi"("error in (no error)"=w238, "quantity"=u16 4, "starting address"=u16 4340, "MB session in"=w243) -> ("error out"=w237:errorcluster, "Registers"=w240:u16[], "MB session out"=w239:refnum<class "MB_Master.lvclass">)  [unwired: 5 in]
        n130 = Insert Into Array(array=w259, new element #1=w258, new element #2=w254, new element #3=w250, new element #4=w245, new element #5=w240) -> (w257:u16[])  [unwired: 1 in]
        n131 = case shown="No Error" w237 {
          tunnel: w257 -> [w274 _]
          frame No Error {
            n132 = call "关键参数区.vi"("数组"=w274) -> ("关键参数区"=w273:T3)  [unwired: 10 in]
            "关键参数区" <- w273
            n133 = global write "VAR挥发酚全局变量.vi" "关键参数区"(w273) -> ()
          }
          frame Error {
          }
        }
      }
      frame "读序列号" {
        n134 = Variant To Data(type=u8 1 ("Slave ID"), Variant=w280) -> (data=w278:u8)  [unwired: 1 in, 1 out]
        n135 = property class="MB_Master"(reference=w283, error in=w284, "Properties:Slave ID"=w278) -> (reference out=w282:refnum<class "MB_Master.lvclass">, error out=w281:errorcluster)
        n136 = call <vilib>:"Read Holding Registers.vi"("error in (no error)"=w281, "quantity"=u16 6, "starting address"=u16 4, "MB session in"=w282) -> ("error out"=w288:errorcluster, "Registers"=w277:u16[], "MB session out"=w287:refnum<class "MB_Master.lvclass">)  [unwired: 5 in]
        n137 = call "HexToString.vi"("数组"=w277) -> ("STRING"=w276:string[])  [unwired: 10 in]
        n138 = Index Array(array=w276) -> (element=w275:string)  [unwired: 1 in]
        "序列号" <- w275
        n139 = global write "VAR挥发酚全局变量.vi" "序列号"(w275) -> ()
      }
      frame "shutdown" {
        n140 = call-dynamic "Close Session.vi"("error in (no error)"=w291, "MB session in"=w289) -> ("error out"=w290:errorcluster)  [unwired: 9 in]
        n141 = Flush Queue(queue=w293) -> (queue out=w292:refnum<queue>)  [unwired: 1 in, 2 out]
        n142 = Release Queue(queue=w292) -> ()  [unwired: 2 in, 3 out]
      }
    }
    n143 = Unbundle By Name(w131) -> ("status"=w127:bool)
    n144 = Not(x=w127) -> (.not. x?=w130:bool)
    "status" <- w130
    n145 = call <vilib>:"Boolean Crossing PtByPt.vi"("direction"=enum16{"either", "false-true", "true-false"}."either", "input"=w127) -> ("crossing"=w128:bool)  [unwired: 1 in]
    n146 = global write "VAR挥发酚全局变量.vi" "通讯状态"(w130) -> ()
    n147 = case shown="True" w128 {
      tunnel: w127 -> [_ _]
      frame False {
      }
      frame True {
      }
    }
  }
  n148 = Release Queue(queue=w6, error in (no error)=w5) -> ()  [unwired: 1 in, 3 out]
